vi "Set Kasli Configuration.vi"(8 "error in (no error)":errorcluster, 11 "Kasli Wrapper 2.0 in":refnum<class "Kasli Wrapper 2.0.lvclass">) -> (0 "error out":errorcluster, 3 "Kasli Wrapper 2.0 out":refnum<class "Kasli Wrapper 2.0.lvclass">)   [LabVIEW 2020, in "TALOS.lvlib" / "Kasli Wrapper 2.0.lvlib" / "Kasli Wrapper 2.0.lvclass"]
uses:
  Kasli Wrapper 2.0.lvclass
  Kasli Wrapper 2.0.lvclass/Kasli Wrapper 2.0.ctl
  Kasli/Kasli.lvclass
  Kasli Wrapper 2.0.lvlib
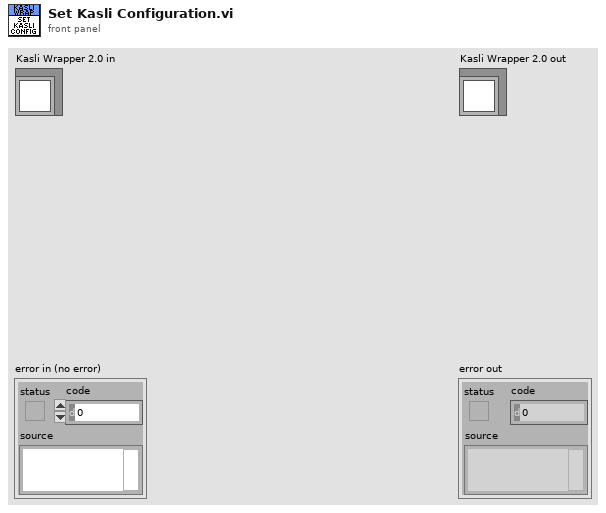
[diagram p1: front panel]
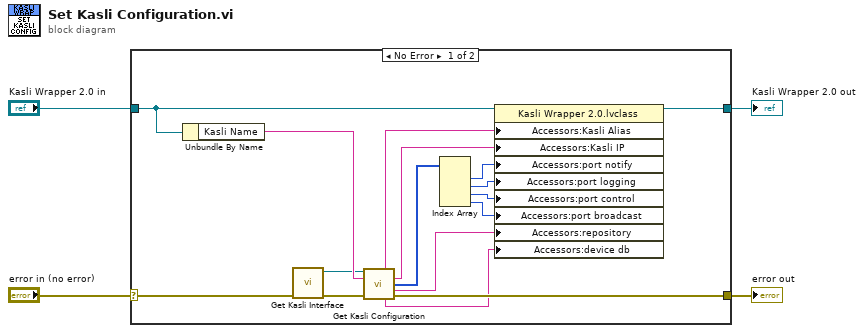
[diagram p0: block diagram]
diagram:
  n1 = case shown="No Error" "error in (no error)" {
    selector: "error in (no error)" -> [w6 w22]
    tunnel: [w20 w22] -> w3
    tunnel: [w8 w21] -> w1
    tunnel: "Kasli Wrapper 2.0 in" -> [w19 w21]
    frame No Error {
      n2 = Unbundle By Name(w19) -> ("Kasli Name"=w18:string)
      n3 = call "Get Kasli Interface.vi"("error in"=w6) -> ("error out"=w5:errorcluster, "Kasli Interface"=w7:refnum<class "Kasli.lvclass">)  [unwired: 9 in]
      n4 = call-dynamic "Get Kasli Configuration.vi"("Kasli in"=w7, "Kasli Name"=w18, "error in (no error)"=w5) -> ("alias"=w16:string, "IP"=w15:string, "ports"=w17:u32[], "repo"=w10:string, "deviceDB"=w9:string, "error out"=w20:errorcluster)  [unwired: 6 in, 1 out]
      n5 = Index Array(array=w17) -> (element #1=w11:u32, element #2=w14:u32, element #3=w13:u32, element #4=w12:u32)  [unwired: 4 in]
      n6 = property class="Kasli Wrapper 2.0.lvclass"(reference=w19, "Accessors:Kasli Alias"=w16, "Accessors:Kasli IP"=w15, "Accessors:port notify"=w11, "Accessors:port logging"=w14, "Accessors:port control"=w13, "Accessors:port broadcast"=w12, "Accessors:repository"=w10, "Accessors:device db"=w9) -> (reference out=w8:refnum<class "Kasli Wrapper 2.0.lvclass">)  [unwired: 1 in, 1 out]
    }
    frame Error {
    }
  }
  "error out" <- w3
  "Kasli Wrapper 2.0 out" <- w1
